vi "try.vi"() -> ()   [LabVIEW 2023]
panel:
  out "Detected":bool
  out "output string":string
  out "error out":errorcluster
  out "return value":string
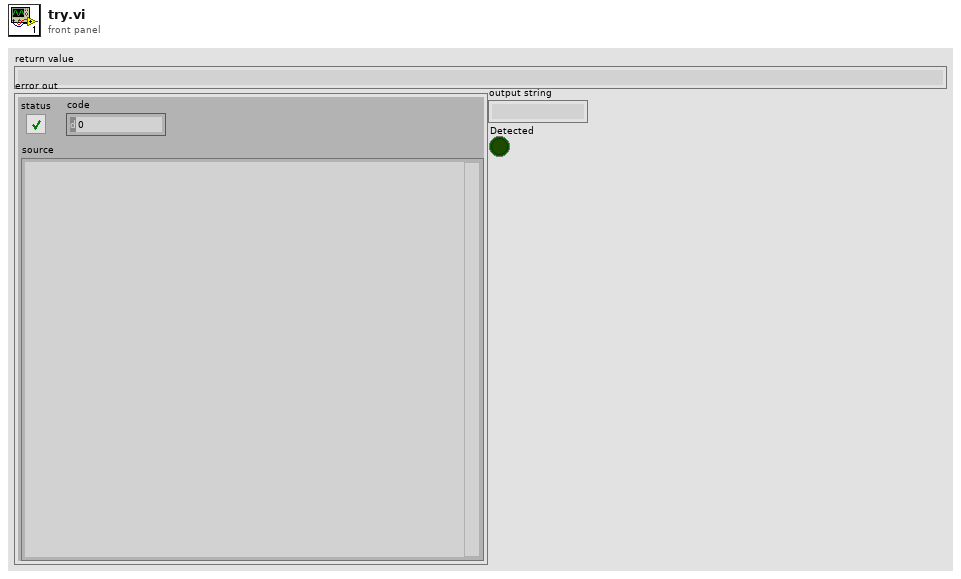
[diagram p1: front panel]
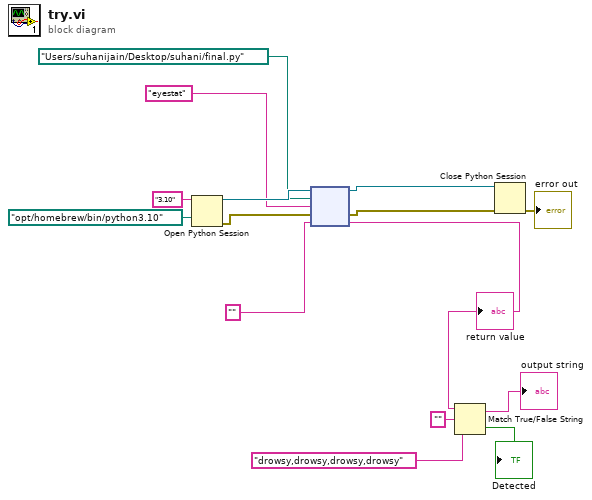
[diagram p0: block diagram]
diagram:
  n1 = Open Python Session(python version="3.10" ("Python version"), python path=path "/opt/homebrew/bin/python3.10" ("Python path")) -> (session out=w14:refnum<k35>, error out=w12:errorcluster)  [unwired: 1 in]
  n2 = node ("Python Node")(w14, path "/Users/suhanijain/Desktop/suhani/final.py" ("module path"), "eyestat" ("Python version"), w12, "" ("Python version")) -> (w13:refnum<k35>, w11:errorcluster, w5:string)  [unwired: 2 out]
  "return value" <- w5
  n3 = Match True/False String(2:"drowsy,drowsy,drowsy,drowsy" ("false string"), 3:"" ("true string"), 4:w5) -> (0:→"Detected":bool, 1:→"output string":string)
  n4 = Close Python Session(session in=w13, error in=w11) -> (11:→"error out":errorcluster)
